vi "P4CMD Get StaticVI Path.vi"() -> (7 "staticVI path":path)   [LabVIEW 2017, in "NI_SCC_P4CMD.lvlib"]
uses:
  <vilib>/SourceControl/Providers/P4CMD/NI_SCC_P4CMD.lvlib
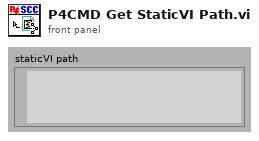
[diagram p1: front panel]
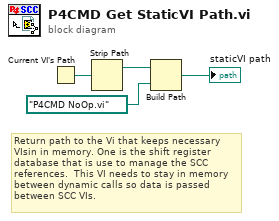
[diagram p0: block diagram]
diagram:
  # "Return path to the Vi that keeps necessary VIsin in memory. One is the shift register database that is use to manage the SCC references.  This VI needs to stay in memory between dynamic calls so data is passed between SCC VIs."
  n1 = Current VI's Path() -> (path=w4:path)
  n2 = Strip Path(path=w4) -> (stripped path=w3:path)  [unwired: 1 out]
  n3 = Build Path(base path=w3, name or relative path=path "P4CMD NoOp.vi") -> (appended path=→"staticVI path":path)
